vi "Run_Slow_Mosaic.vi"(2 "Take Snap \narray":u64[](array[numeric])=[0, 0, 0, 0, 0, 0, 0, 0, 0, 0, 0, 0, 0, 0, 0, 0, 0, 0, 0, 0, 0, 0, 0, 0, 0, 0, 0, 0, 0, 0, 0, 0, 0, 0, 0, 0, 0, 0, 0, 0, 0, 0, 0, 0, 0, 0, 0, 0, 0, 0], 3 "Mosaic Size":fxp<+,6,6>) -> (0 "Error Out":u8, 1 "Aborted":bool)   [LabVIEW 2024]
uses:
  <vilib>/rvi/eio/common/nirviEmuTemplateMethod_errors.vi
  <vilib>/rvi/Emulation/niFpgaGetClockAttributes.vi
  <vilib>/rvi/Emulation/niFpgaSctlEmulationGetInTimedLoop.vi
  <vilib>/rvi/Emulation/niFpgaEmulationReportErrorSimple.vi
  <vilib>/rvi/Emulation/niFpgaCriticalErrorInLSC.vi
  <vilib>/eio/EIONode/EIONode.xnode
  <vilib>/eio/EIOMethodNode/EIOMethodNode.xnode
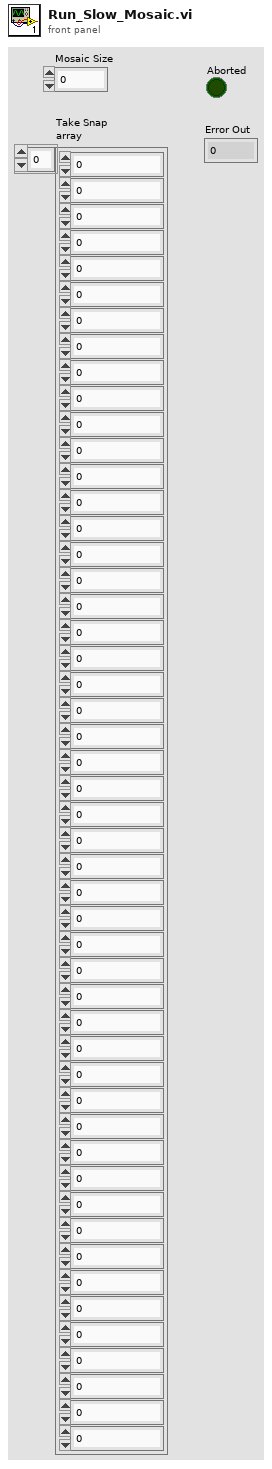
[diagram p1: front panel]
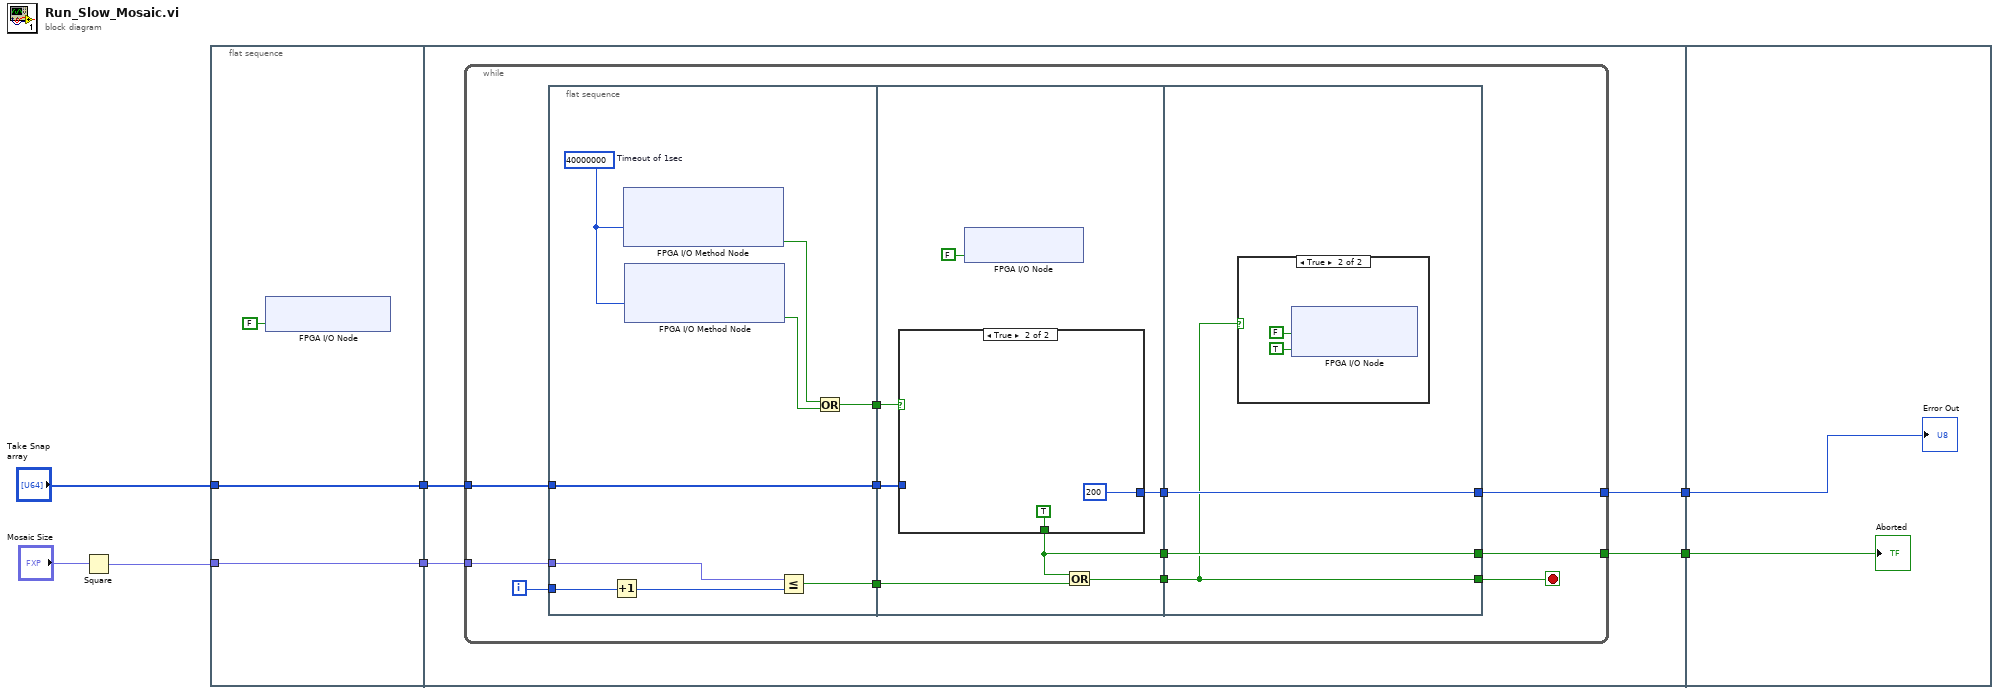
[diagram p0: block diagram]
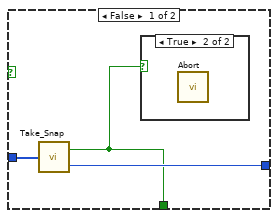
[diagram p2: hidden frame]
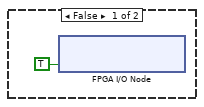
[diagram p4: hidden frame]
diagram:
  n1 = Square(x="Mosaic Size") -> (x^2=w3:fxp<+,12,12>)
  n2 = flat-sequence {
    tunnel: "Take Snap \narray" -> [w9]
    tunnel: w3 -> [w10]
    tunnel: [w10] -> w2
    tunnel: [w9] -> w1
    tunnel: [w14] -> w7
    tunnel: [w12] -> w4
    tunnel: w2 -> [w11]
    tunnel: w1 -> [w13]
    tunnel: w7 -> [w55]
    tunnel: w4 -> [w54]
    frame #0 {
      n3 = xnode "FPGA I/O Node"("Stage Abort OUT"=FALSE) -> ()  [unwired: 1 in, 1 out]
    }
    frame #1 {
      n4 = while {
        tunnel: [w18] -> w14
        tunnel: w13 -> [w25]
        tunnel: [w24] -> w12
        tunnel: w11 -> [w21]
        i -> [w22]
        stop <- w17 stop-if-true
        n5 = flat-sequence {
          tunnel: [w35] -> w26
          tunnel: w25 -> [w35]
          tunnel: w22 -> [w33]
          tunnel: w21 -> [w32]
          tunnel: [w31] -> w20
          tunnel: [w27] -> w15
          tunnel: w26 -> [w42]
          tunnel: [w41] -> w23
          tunnel: w20 -> [w39]
          tunnel: [w38] -> w19
          tunnel: [w37] -> w16
          tunnel: w15 -> [w36]
          tunnel: [w50] -> w24
          tunnel: w23 -> [w50]
          tunnel: w19 -> [w49]
          tunnel: [w49] -> w18
          tunnel: [w48] -> w17
          tunnel: w16 -> [w48]
          frame #0 {
            w30 = 40000000  # Timeout of 1sec
            n6 = Increment(x=w33) -> (x+1=w34:i32)
            n7 = xnode "FPGA I/O Method Node"("Timeout"=w30) -> ("Timed Out"=w29:bool)  [unwired: 1 in, 1 out]
            n8 = xnode "FPGA I/O Method Node"("Timeout"=w30) -> ("Timed Out"=w28:bool)  [unwired: 1 in, 1 out]
            n9 = Less Or Equal?(x=w32, y=w34) -> (x <= y?=w31:bool)
            n10 = Or(x=w29, y=w28) -> (x .or. y?=w27:bool)
          }
          frame #1 {
            n11 = case shown="True" w36 {
              tunnel: w42 -> [w45 _]
              tunnel: [w44 u8 200 ("Error Out")] -> w41
              tunnel: [w43 TRUE ("Aborted")] -> w38
              frame False {
                n12 = call "Take_Snap.vi"("Take Snap \narray"=w45) -> ("Aborted"=w43:bool, "Error Out"=w44:u8)
                n13 = case shown="True" w43 {
                  frame False {
                  }
                  frame True {
                    n14 = call "Abort.vi"() -> ()  [unwired: 12 in]
                  }
                }
              }
              frame True {
              }
            }
            n15 = xnode "FPGA I/O Node"("Stage Next OUT"=FALSE ("Idle OUT")) -> ()  [unwired: 1 in, 1 out]
            n16 = Or(x=w38, y=w39) -> (x .or. y?=w37:bool)
          }
          frame #2 {
            n17 = case shown="True" w48 {
              frame False {
                n18 = xnode "FPGA I/O Node"("Stage Next OUT"=TRUE ("Idle OUT")) -> ()  [unwired: 1 in, 1 out]
              }
              frame True {
                n19 = xnode "FPGA I/O Node"("Stage Next OUT"=FALSE ("Idle OUT"), "Stage Abort OUT"=TRUE ("Stage Abort")) -> ()  [unwired: 2 in, 2 out]
              }
            }
          }
        }
      }
    }
    frame #2 {
      "Aborted" <- w55
      "Error Out" <- w54
    }
  }
